vi "PAQmem_ReadRecent.vi"(8 "error in (no error)":errorcluster, 9 "TimeSpan(sec)":dbl, 10 "TagsIndices":i32[](array[numeric]), 11 "PAQ-memory in":refnum<class "PAQ-memory.lvclass">) -> (0 "error out":errorcluster, 2 "PAQ_section":T1, 3 "PAQ-memory out":refnum<class "PAQ-memory.lvclass">)   [LabVIEW 2020, in "Sgraph_lib_V1.lvlib" / "PAQ-memory.lvclass"]
doc: "Andre Koelewijn, 17 Jan 2021\n\nRead from PAQ memory at the end (latest data) of the buffer"
uses:
  PAQ-memory.lvclass
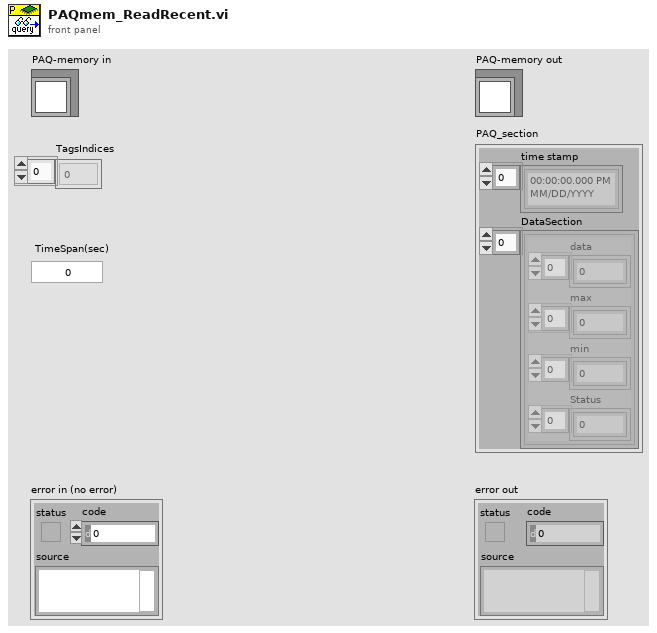
[diagram p1: front panel]
types:
  T1 = cluster{"time stamp":timestamp[], "DataSection":cluster{"data":dbl[], "max":dbl[], "min":dbl[], "Status":u32[]}[]}
  T2 = cluster{"data":dbl[], "max":dbl[], "min":dbl[], "Status":u32[]}[]
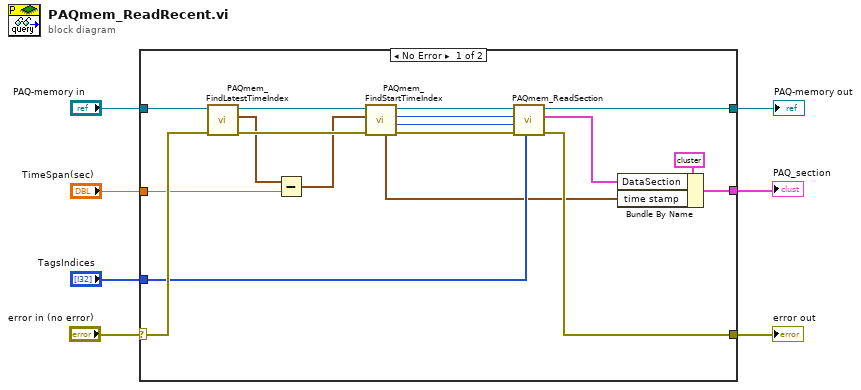
[diagram p0: block diagram]
diagram:
  n1 = case shown="No Error" "error in (no error)" {
    selector: "error in (no error)" -> [w23 w27]
    tunnel: [w13 w27] -> w6
    tunnel: [w17 w26] -> w4
    tunnel: "PAQ-memory in" -> [w24 w26]
    tunnel: "TimeSpan(sec)" -> [w20 _]
    tunnel: "TagsIndices" -> [w12 _]
    tunnel: [w8 _] -> w1
    frame No Error {
      n2 = call "PAQmem_FindLatestTimeIndex.vi"("error in (no error)"=w23, "PAQ-memory in"=w24) -> ("error out"=w22:errorcluster, "Time"=w21:timestamp, "PAQ-memory out"=w25:refnum<class "PAQ-memory.lvclass">)  [unwired: 6 in, 1 out]
      n3 = Subtract(x=w21, y=w20) -> (x-y=w19:timestamp)
      n4 = call "PAQmem_FindStartTimeIndex.vi"("error in (no error)"=w22, "Start-time"=w19, "PAQ-memory in"=w25) -> ("error out"=w14:errorcluster, "Size"=w15:i32, "Start"=w16:i32, "PAQ-memory out"=w18:refnum<class "PAQ-memory.lvclass">, "time"=w9:timestamp[])  [unwired: 4 in]
      n5 = call "PAQmem_ReadSection.vi"("TagsIndices"=w12, "error in (no error)"=w14, "Length"=w15, "Start"=w16, "PAQ-memory in"=w18) -> ("error out"=w13:errorcluster, "DataSection"=w10:T2, "PAQ-memory out"=w17:refnum<class "PAQ-memory.lvclass">)  [unwired: 4 in]
      n6 = Bundle By Name(cluster=T1 {"time stamp"=[timestamp(3693737062.1268244 s since 1904-01-01), timestamp(3693737063.0693784 s since 1904-01-01), timestamp(3693737064.0694356 s since 1904-01-01), timestamp(3693737065.069493 s since 1904-01-01), timestamp(3693737066.0695496 s since 1904-01-01), timestamp(3693737067.0696073 s since 1904-01-01), timestamp(3693737068.069664 s since 1904-01-01), timestamp(3693737069.069721 s since 1904-01-01), timestamp(3693737070.0697784 s since 1904-01-01), timestamp(3693737071.069836 s since 1904-01-01), timestamp(3693737072.069893 s since 1904-01-01), timestamp(3693737073.0694504 s since 1904-01-01), timestamp(3693737074.069008 s since 1904-01-01), timestamp(3693737075.0690646 s since 1904-01-01), timestamp(3693737076.0691223 s since 1904-01-01), timestamp(3693737077.0691795 s since 1904-01-01), timestamp(3693737078.0692368 s since 1904-01-01), timestamp(3693737079.0692935 s since 1904-01-01), timestamp(3693737080.069351 s since 1904-01-01), timestamp(3693737081.069408 s since 1904-01-01), timestamp(3693737082.0694656 s since 1904-01-01), timestamp(3693737083.069522 s since 1904-01-01), timestamp(3693737084.0695796 s since 1904-01-01), timestamp(3693737085.069637 s since 1904-01-01), timestamp(3693737086.0696936 s since 1904-01-01), timestamp(3693737087.069751 s since 1904-01-01), timestamp(3693737088.069808 s since 1904-01-01), timestamp(3693737089.069865 s since 1904-01-01), timestamp(3693737090.0699224 s since 1904-01-01), timestamp(3693737091.06948 s since 1904-01-01), timestamp(3693737092.069037 s since 1904-01-01), timestamp(3693737093.069094 s since 1904-01-01), timestamp(3693737094.069152 s since 1904-01-01), timestamp(3693737095.0692086 s since 1904-01-01), timestamp(3693737096.069266 s since 1904-01-01), timestamp(3693737097.069323 s since 1904-01-01), timestamp(3693737098.0693808 s since 1904-01-01), timestamp(3693737099.0694375 s since 1904-01-01), timestamp(3693737100.0694947 s since 1904-01-01), timestamp(3693737101.0695515 s since 1904-01-01), timestamp(3693737102.0696096 s since 1904-01-01), timestamp(3693737103.069666 s since 1904-01-01), timestamp(3693737104.069723 s since 1904-01-01), timestamp(3693737105.0697803 s since 1904-01-01), timestamp(3693737106.0698376 s since 1904-01-01), timestamp(3693737107.069895 s since 1904-01-01), timestamp(3693737108.0694523 s since 1904-01-01), timestamp(3693737109.0690093 s since 1904-01-01), timestamp(3693737110.069067 s since 1904-01-01), timestamp(3693737111.0691237 s since 1904-01-01), timestamp(3693737112.069181 s since 1904-01-01), timestamp(3693737113.069238 s since 1904-01-01), timestamp(3693737114.069296 s since 1904-01-01), timestamp(3693737115.0693526 s since 1904-01-01), timestamp(3693737116.06941 s since 1904-01-01), timestamp(3693737117.069467 s since 1904-01-01), timestamp(3693737118.069525 s since 1904-01-01), timestamp(3693737119.0695815 s since 1904-01-01), timestamp(3693737120.0696387 s since 1904-01-01), timestamp(3693737121.072196 s since 1904-01-01), timestamp(3693737122.0747533 s since 1904-01-01), timestamp(3693737123.0748105 s since 1904-01-01)], "DataSection"=[]} ("PAQ_section"), "DataSection"=w10, "time stamp"=w9) -> (w8:T1)
    }
    frame Error {
    }
  }
  "error out" <- w6
  "PAQ-memory out" <- w4
  "PAQ_section" <- w1
